vi "Exercise1.6-Waveform.vi"() -> ()   [LabVIEW 2013]
panel:
  out "output waveform":waveform(dbl)
  out "Y":dbl[](array[numeric])
  out "dt":dbl
  out "t0":timestamp
  in  "waveform":waveform(dbl)
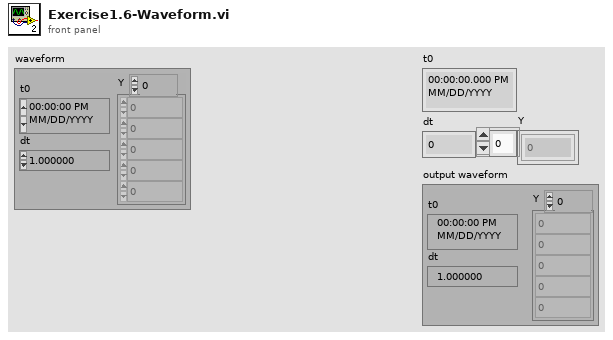
[diagram p1: front panel]
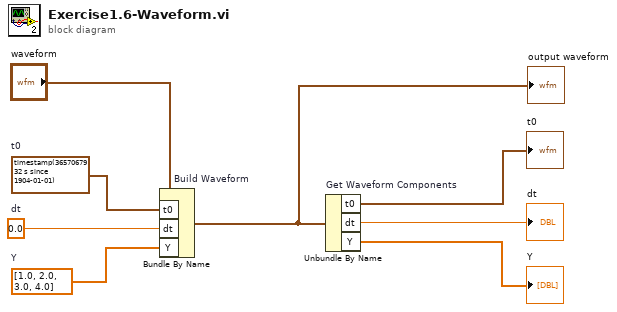
[diagram p0: block diagram]
diagram:
  w5 = dbl[] [1.0, 2.0, 3.0, 4.0]  # Y
  w6 = 0.0  # dt
  w7 = timestamp(3657067932 s since 1904-01-01)  # t0
  n1 = Bundle By Name "Build Waveform"(cluster="waveform", "t0"=w7, "dt"=w6, "Y"=w5) -> (w4:waveform(dbl))
  "output waveform" <- w4
  n2 = Unbundle By Name "Get Waveform Components"(w4) -> ("t0"=→"t0":timestamp, "dt"=→"dt":dbl, "Y"=→"Y":dbl[])
